vi "connect to command stream.vi"(9 "Queues":T1, 11 "comms in":T2) -> (3 "comms out":T2)   [LabVIEW 2018]
uses:
  type defs/comms loop data.ctl
  Github/ICL-LabVIEW_General/Incident logger/Incident logger.lvclass
  <vilib>/Modbus/master/Modbus Master.lvclass
  type defs/Queues.ctl
  supporting VIs/polymorphic VIs/enqueue for comms.vi
  supporting VIs/polymorphic VIs/enqueue for message handler.vi
types:
  T1 = typedef "Queues.ctl" = cluster{"messageHandler":refnum<queue>, "comms":refnum<queue>, "dataStream":refnum<queue>, "dataProcessor":refnum<queue>, "fileIO":refnum<queue>, "userInterface":refnum<queue>, "errors":refnum<queue>, "customCompressor":refnum<queue>}
  T2 = typedef "comms loop data.ctl" = cluster{"params":cluster{"commandStream":cluster{"reader name":string, "writer name":string, "stream buffer size":i32}, "errorStream":cluster{"reader name":string, "writer name":string, "stream buffer size":i32}, "RT IP address":string, "pulserControllerIP":string}, "vars":cluster{"commandStream":refnum<k21>, "Incident logger":refnum<class "Incident logger.lvclass">, "check error scheduled message":u32, "errorStream":refnum<k21>, "watchdogScheduleID":u32, "pulsator":cluster{"pulser connection":refnum<class "Modbus Master.lvclass">, "pulserConnected":bool, "pulsatorScheduleID":u32, "pulserRunning":bool}}}
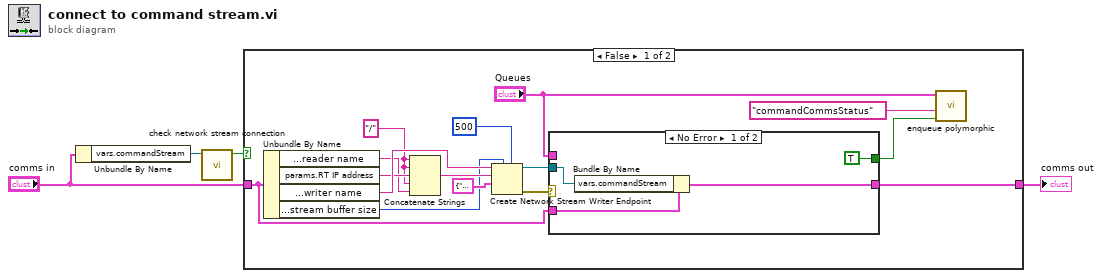
[diagram p0: block diagram]
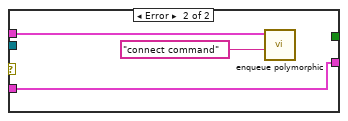
[diagram p2: hidden frame]
diagram:
  n1 = Unbundle By Name("comms in") -> ("vars.commandStream"=w4:refnum<k21>)
  n2 = call "check network stream connection.vi"("stream ref"=w4) -> ("Connected"=w3:bool)  [unwired: 10 in]
  n3 = case shown="False" w3 {
    tunnel: "comms in" -> [w8 w27]
    tunnel: [w9 w27] -> w1
    frame False {
      w17 = "/" ("string")
      n4 = Unbundle By Name(w8) -> ("params.commandStream.reader name"=w16:string, "params.RT IP address"=w18:string, "params.commandStream.writer name"=w19:string, "params.commandStream.stream buffer size"=w13:i32)
      n5 = Concatenate Strings(w17, w17, w18, w17, w16) -> (w15:string)
      n6 = Create Network Stream Writer Endpoint(5:500 ("timeout in ms (-1)"), 7:w13, 9:cluster{"message":string, "data":variant} {"message"="", "data"=variant}, 10:w15, 11:w19) -> (0:w11:errorcluster, 3:w10:refnum<k21>)  [unwired: 2 in]
      n7 = case shown="No Error" w11 {
        tunnel: w10 -> [w22 _]
        tunnel: w8 -> [w21 w26]
        tunnel: [w23 w26] -> w9
        tunnel: "Queues" -> [_ w24]
        tunnel: [TRUE ("Boolean") _] -> w6
        frame No Error {
          n8 = Bundle By Name(cluster=w21, "vars.commandStream"=w22) -> (w23:T2)
        }
        frame Error {
          n9 = call-poly "enqueue polymorphic.vi"("message"="connect command", "Queues"=w24) -> ()  [unwired: 9 in, 1 out]
        }
      }
      n10 = call-poly "enqueue polymorphic.vi"("data"=w6, "message"="commandCommsStatus", "Queues"="Queues") -> ()  [unwired: 8 in, 1 out]
    }
    frame True {
    }
  }
  "comms out" <- w1
